vi "Change Configuration Attributes While Acquiring.vi"() -> ()   [LabVIEW 2023]
doc: "The Change Configuration Attributes While Acquiring example acquires images continuously and demonstrates how to set attributes that are not writeable while acquiring by stopping and unconfiguring the acquisition before writing these attributes."
uses:
  <vilib>/vision/driver/NI_Vision_Acquisition_Software.lvlib
  <resource>/objmgr/imaqdx.rc
panel:
  out "Attribute Writeable":bool
  out "Acquisition in Progress":bool
  out "Frame Rate":dbl
  in  "Camera Name":refnum<k21> caption="IMAQdx Session"
  in  "Image Size Parameters":cluster{"Width":u32, "Height":u32}={"Width"=8, "Height"=8} {"Height" min=1 max=32768 step=1; "Width" min=1 max=32768 step=1}
  out "Buffer Number":u32
  out "Image":T1(plugin-control)
  in  "Stop":bool
  # "Overview: Demonstrates how to modify the Image Size Parameters while acquiring a continuous acquisition.\nRequirements: Vision Acquisition Software.\nInstructions: \n1. Select the Camera Name\n2. Run the VI\n3. Modify the Image Size Parameters."
  # "Note: The attributes aren't writeable while acquiring. This example stops the acquisition to write these attributes."
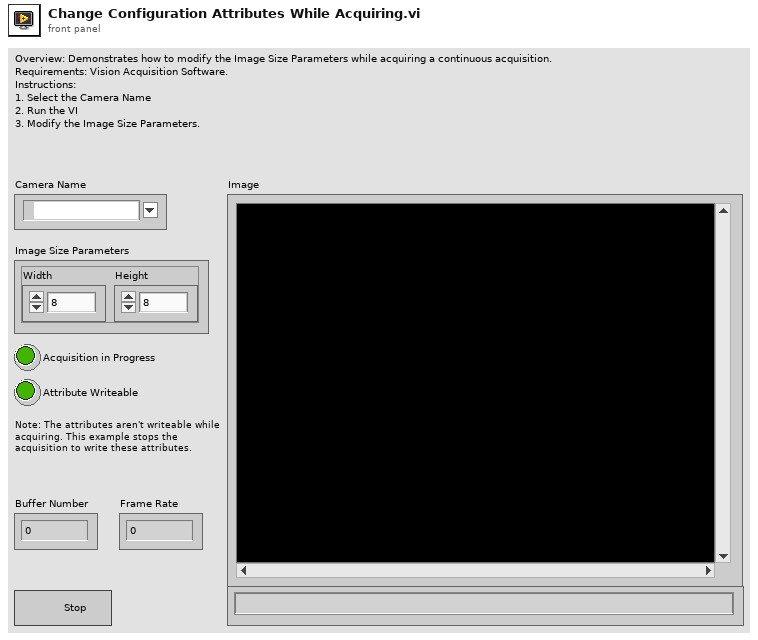
[diagram p1: front panel]
types:
  T1 = typedef "IMAQ Image.ctl" = refnum<image>
  T2 = typedef "IMAQdx.ctl" = refnum<k21>
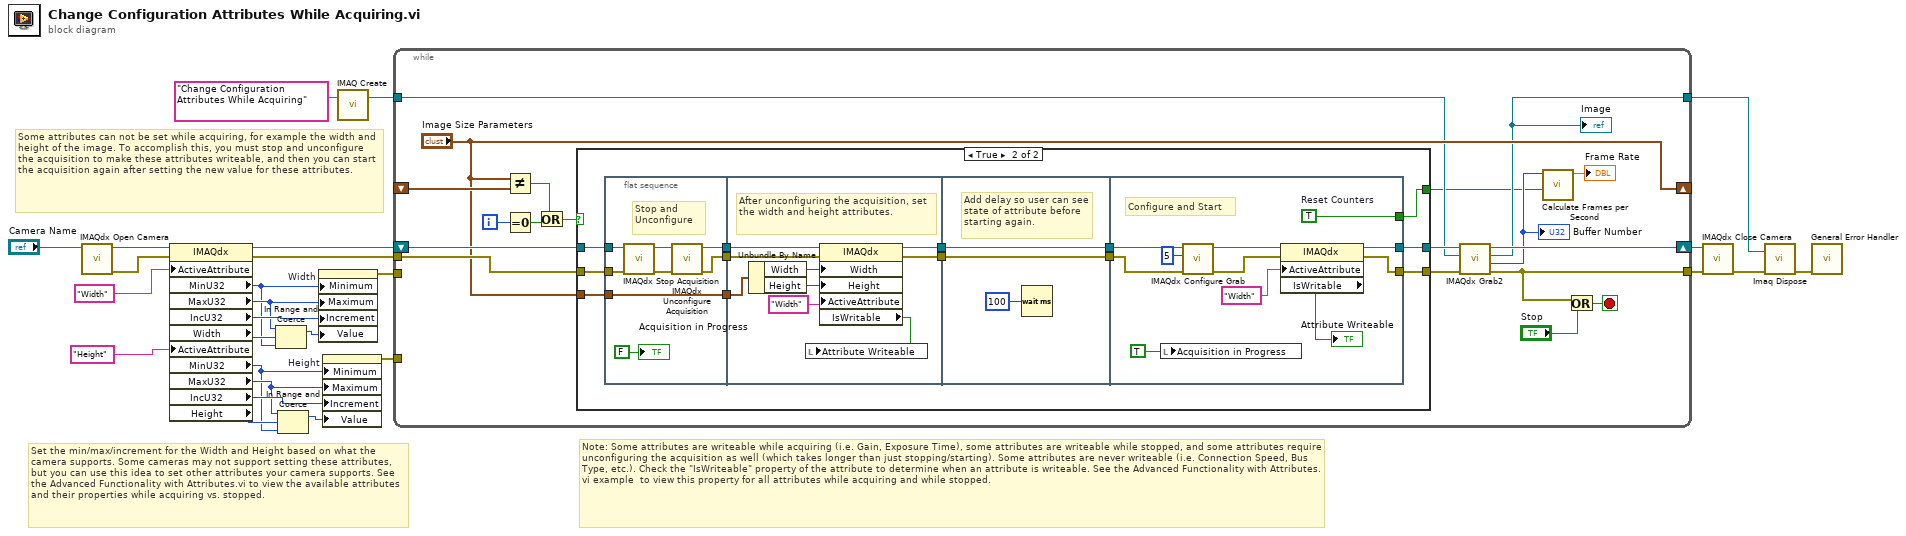
[diagram p0: block diagram]
diagram:
  # "Set the min/max/increment for the Width and Height based on what the camera supports. Some cameras may not support setting these attributes, but you can use this idea to set other attributes your camera supports. See the Advanced Functionality with Attributes.vi to view the available attributes and their properties while acquiring vs. stopped."
  # "Note: Some attributes are writeable while acquiring (i.e. Gain, Exposure Time), some attributes are writeable while stopped, and some attributes require unconfiguring the acquisition as well (which takes longer than just stopping/starting). Some attributes are never writeable (i.e. Connection Speed, Bus Type, etc.). Check the \"IsWriteable\" property of the attribute to determine when an attribute is writeable. See the Advanced Functionality with Attributes.vi example  to view this property for all attributes while acquiring and while stopped."
  # "Some attributes can not be set while acquiring, for example the width and height of the image. To accomplish this, you must stop and unconfigure the acquisition to make these attributes writeable, and then you can start the acquisition again after setting the new value for these attributes."
  n1 = call <vilib>:"IMAQdx Open Camera.vi"("Session In"="Camera Name") -> ("error out"=w16:errorcluster, "Session Out"=w18:T2)  [unwired: 2 in, 7 out]
  n2 = property class="IMAQdx"(reference=w18, error in=w16, "ActiveAttribute"="Width", "ActiveAttribute"="Height") -> (reference out=w17:T2, error out=w9:errorcluster, "MinU32"=w11:u32, "MaxU32"=w12:u32, "IncU32"=w14:u32, "Width"=w13:u32, "MinU32"=w4:u32, "MaxU32"=w5:u32, "IncU32"=w7:u32, "Height"=w6:u32)
  n3 = In Range and Coerce(upper limit=w12, x=w13, lower limit=w11) -> (coerced(x)=w10:u32)  [unwired: 1 out]
  n4 = In Range and Coerce(upper limit=w5, x=w6, lower limit=w4) -> (coerced(x)=w3:u32)  [unwired: 1 out]
  n5 = property on="Width" class="DigNum (strict)"("Minimum"=w11, "Maximum"=w12, "Increment"=w14, "Value"=w10) -> (error out=w1:errorcluster)  [unwired: 2 in, 1 out]
  n6 = property on="Height" class="DigNum (strict)"("Minimum"=w4, "Maximum"=w5, "Increment"=w7, "Value"=w3) -> (error out=w2:errorcluster)  [unwired: 2 in, 1 out]
  n7 = call "IMAQ Create"("Image Name"="Change Configuration Attributes While Acquiring") -> ("New Image"=w26:T1)  [unwired: 3 in, 2 out]
  n8 = while {
    tunnel: [w31] -> w24
    tunnel: w26 -> [w30]
    shift-right: ["Image Size Parameters"] -> _
    shift-left: _ -> [w38]
    tunnel: w9 -> [w39]
    shift-right: [w43] -> w25
    shift-left: w17 -> [w40]
    tunnel: [w29] -> w21
    tunnel: w2 -> [_]
    tunnel: w1 -> [_]
    i -> [w32]
    stop <- w45 stop-if-true
    n9 = Not Equal?(x="Image Size Parameters", y=w38) -> (x != y?=w34:bool)
    n10 = Equal To 0?(x=w32) -> (x = 0?=w37:bool)
    n11 = Or(x=w34, y=w37) -> (x .or. y?=w36:bool)
    n12 = case shown="True" w36 {
      tunnel: [w46 w48] -> w42
      tunnel: [w47 w49] -> w41
      tunnel: w40 -> [w47 w60]
      tunnel: w39 -> [w46 w59]
      tunnel: "Image Size Parameters" -> [_ w55]
      tunnel: [_ w50] -> w27
      frame False {
      }
      frame True {
        n13 = flat-sequence {
          tunnel: w60 -> [w64]
          tunnel: w59 -> [w63]
          tunnel: [w68] -> w58
          tunnel: [w67] -> w57
          tunnel: [w65] -> w56
          tunnel: w55 -> [w65]
          tunnel: w58 -> [w73]
          tunnel: w57 -> [w72]
          tunnel: w56 -> [w71]
          tunnel: [w70] -> w54
          tunnel: [w69] -> w52
          tunnel: w54 -> [w80]
          tunnel: [w80] -> w53
          tunnel: w52 -> [w79]
          tunnel: [w79] -> w51
          tunnel: w53 -> [w85]
          tunnel: w51 -> [w84]
          tunnel: [w90] -> w50
          tunnel: [w89] -> w49
          tunnel: [w88] -> w48
          frame #0 {
            # "Stop and Unconfigure"
            n14 = call <vilib>:"IMAQdx Stop Acquisition.vi"("error in"=w63, "Session In"=w64) -> ("error out"=w62:errorcluster, "Session Out"=w61:T2)  [unwired: 8 in]
            n15 = call <vilib>:"IMAQdx Unconfigure Acquisition.vi"("error in"=w62, "Session In"=w61) -> ("error out"=w67:errorcluster, "Session Out"=w68:T2)  [unwired: 8 out]
            "Acquisition in Progress" <- FALSE ("Acquiring")
          }
          frame #1 {
            # "After unconfiguring the acquisition, set the width and height attributes."
            n16 = Unbundle By Name(w71) -> ("Width"=w77:u32, "Height"=w76:u32)
            n17 = property class="IMAQdx"(reference=w73, error in=w72, "Width"=w77, "Height"=w76, "ActiveAttribute"="Width") -> (reference out=w70:T2, error out=w69:errorcluster, "IsWritable"=w74:bool)
            n18 = local write "Attribute Writeable"(w74) -> ()
          }
          frame #2 {
            # "Add delay so user can see state of attribute before starting again."
            n19 = Wait (ms)(milliseconds to wait=u32 100) -> ()  [unwired: 1 out]
          }
          frame #3 {
            w90 = TRUE  # Reset Counters
            # "Configure and Start"
            n20 = local write "Acquisition in Progress"(TRUE ("Acquiring")) -> ()
            n21 = call <vilib>:"IMAQdx Configure Grab.vi"("error in"=w84, "Number of Buffers"=u32 5, "Session In"=w85) -> ("error out"=w83:errorcluster, "Session Out"=w82:T2)  [unwired: 7 in]
            n22 = property class="IMAQdx"(reference=w82, error in=w83, "ActiveAttribute"="Width") -> (reference out=w89:T2, error out=w88:errorcluster, "IsWritable"=→"Attribute Writeable":bool)
          }
        }
      }
    }
    n23 = call <vilib>:"IMAQdx Grab2.vi"("error in"=w42, "Image In"=w30, "Session In"=w41) -> ("error out"=w31:errorcluster, "Buffer Number Out"=w35:u32, "Image Out"=w29:T1, "Session Out"=w43:T2)  [unwired: 5 in]
    "Image" <- w29
    "Buffer Number" <- w35
    n24 = call <vilib>:"Calculate Frames per Second.vi"("Reset"=w27, "Buffer Number"=w35) -> ("Acquired Frames/s"=→"Frame Rate":dbl)  [unwired: 7 in, 2 out]
    n25 = Or(x=w31, y="Stop") -> (x .or. y?=w45:bool)
  }
  n26 = call <vilib>:"IMAQdx Close Camera.vi"("error in"=w24, "Session In"=w25) -> ("error out"=w23:errorcluster)  [unwired: 9 out]
  n27 = call "Imaq Dispose"("Image"=w21, "error in (no error)"=w23) -> ("error out"=w22:errorcluster)  [unwired: 4 in]
  n28 = call <vilib>:"General Error Handler.vi"("error in (no error)"=w22) -> ()  [unwired: 2 in, 13 out]
